vi "SaveOk.vi"() -> ()   [LabVIEW 2019]
panel:
  in  "OK Button":bool
  # "Zapisywanie zakoñczone"
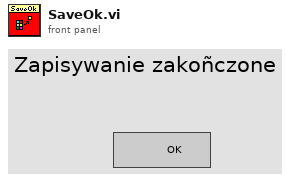
[diagram p1: front panel]
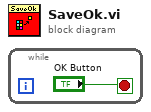
[diagram p0: block diagram]
diagram:
  n1 = while {
    stop <- "OK Button" stop-if-true
  }
